vi "RunOperation.vi"(10 "Inputs":string[](array[string]), 11 "RunTests in":refnum<class "RunVITester.lvclass">) -> (1 "Output/Failure":string, 2 "CLI Process Return Code":i32, 3 "RunTests out":refnum<class "RunVITester.lvclass">)   [LabVIEW 2027, in "RunVITester.lvclass"]
uses:
  RunVITester.lvclass
  <vilib>/addons/_JKI.lib/_jki_lib_vi_tester_junit_xml_results.llb/TextTestRunner.JUnitXML.lvclass
  RunVITester.lvclass/RunVITester.ctl
  <vilib>/addons/_JKI Toolkits/VI Tester/VI Tester API.llb/Run Tests (Path Array).vi
  <vilib>/addons/_JKI Toolkits/VI Tester/VI Tester API.llb/VI Tester API.lvlib
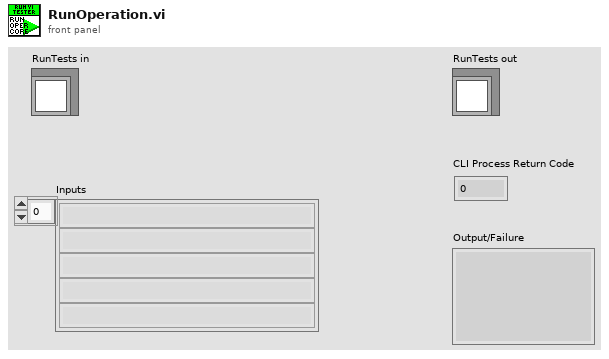
[diagram p1: front panel]
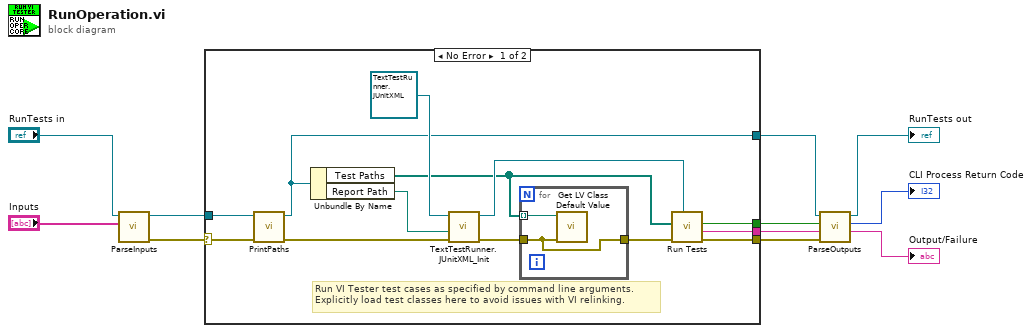
[diagram p0: block diagram]
diagram:
  n1 = call "ParseInputs.vi"("Inputs"="Inputs", "RunTests in"="RunTests in") -> ("error out"=w9:errorcluster, "RunTests out"=w1:refnum<class "RunVITester.lvclass">)  [unwired: 8 in]
  n2 = case shown="No Error" w9 {
    selector: w9 -> [w18 w28]
    tunnel: [w21 w28] -> w8
    tunnel: [w16 w27] -> w5
    tunnel: [w20 _] -> w3
    tunnel: [w19 _] -> w2
    tunnel: w1 -> [w15 w27]
    frame No Error {
      # "Run VI Tester test cases as specified by command line arguments.\nExplicitly load test classes here to avoid issues with VI relinking."
      n3 = call "PrintPaths.vi"("error in (no error)"=w18, "RunVITester in"=w15) -> ("error out"=w17:errorcluster, "RunVITester out"=w16:refnum<class "RunVITester.lvclass">)  [unwired: 8 in]
      n4 = Unbundle By Name(w16) -> ("Test Paths"=w13:path[], "Report Path"=w22:path)
      n5 = call <vilib>:"TextTestRunner.JUnitXML_Init.vi"("error in (no error)"=w17, "Report Path"=w22, "TextTestRunner in"=refnum<class "TextTestRunner.JUnitXML.lvclass"> refnum) -> ("error out"=w14:errorcluster, "TextTestRunner out"=w23:refnum<class "TextTestRunner.JUnitXML.lvclass">)  [unwired: 7 in]
      n6 = for {
        tunnel: w14 -> [w25]
        tunnel: w13 -> [w26] mode=indexing
        tunnel: [w25] -> w12
        n7 = call <vilib>:"Get LV Class Default Value.vi"("error in (no error)"=w25, "class path"=w26) -> ()  [unwired: 8 in, 2 out]
      }
      n8 = call-poly <vilib>:"Run Tests.vi"("TextTestRunner in"=w23, "error in (no error)"=w12, "Test Paths"=w13) -> ("error out"=w21:errorcluster, "test details"=w19:string, "successful?"=w20:bool)  [unwired: 6 in]
    }
    frame Error {
    }
  }
  n9 = call "ParseOutputs.vi"("error in (no error)"=w8, "test details"=w2, "successful?"=w3, "RunTests in"=w5) -> ("Output/Failure"=→"Output/Failure":string, "CLI Process Return Code"=→"CLI Process Return Code":i32, "RunTests out"=→"RunTests out":refnum<class "RunVITester.lvclass">)  [unwired: 4 in, 1 out]
